vi "RecvTCPString.vi"(8 "error in":errorcluster, 11 "TCP Network Connection in":refnum<k5>) -> (0 "error out":errorcluster, 3 "data out":string)   [LabVIEW 2019]
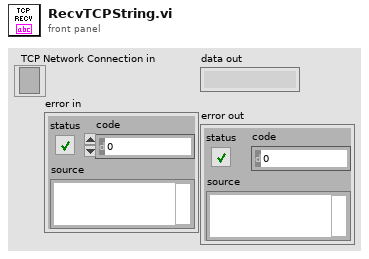
[diagram p1: front panel]
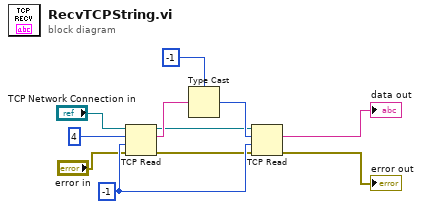
[diagram p0: block diagram]
diagram:
  w6 = -1
  n1 = TCP Read(connection ID="TCP Network Connection in", bytes to read=4, error in (no error)="error in", 9:w6) -> (connection ID out=w4:refnum<k5>, data out=w5:string, error out=w3:errorcluster)  [unwired: 1 in]
  n2 = Type Cast(type=-1, x=w5) -> (*(type *) &x=w10:i32)
  n3 = TCP Read(connection ID=w4, bytes to read=w10, error in (no error)=w3, 9:w6) -> (data out=→"data out":string, error out=→"error out":errorcluster)  [unwired: 1 in, 1 out]
